vi "transition.vi"(0 "new picture in":picture, 3 "state change":bool=TRUE, 4 "game state":T1(ring), 5 "timer":dbl) -> (14 "new picture out":picture, 17 "change (of) scene":bool)   [LabVIEW 2023]
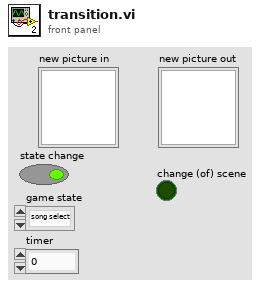
[diagram p1: front panel]
types:
  T1 = enum16{"song select", "difficulty select", "gameplay", "result"}
  T2 = cluster{"horizontal":enum16{"left", "center", "right"}, "vertical":enum16{"top", "center", "bottom"}}
  T3 = cluster{"Font Name:":string, "Size":i16, "Strikeout?":bool, "Italic?":bool, "Underline?":bool, "Outline?":bool, "Shadow?":bool, "Bold?":bool}
  T4 = enum16{"User-specified Font", "Application Font", "System Font", "Dialog Font"}
  T5 = typedef "imagedata.ctl" = cluster{"image type":i32, "image depth":i32, "image":u8[], "mask":u8[], "colors":u32[], "Rectangle":cluster{"left":i16, "top":i16, "right":i16, "bottom":i16}}
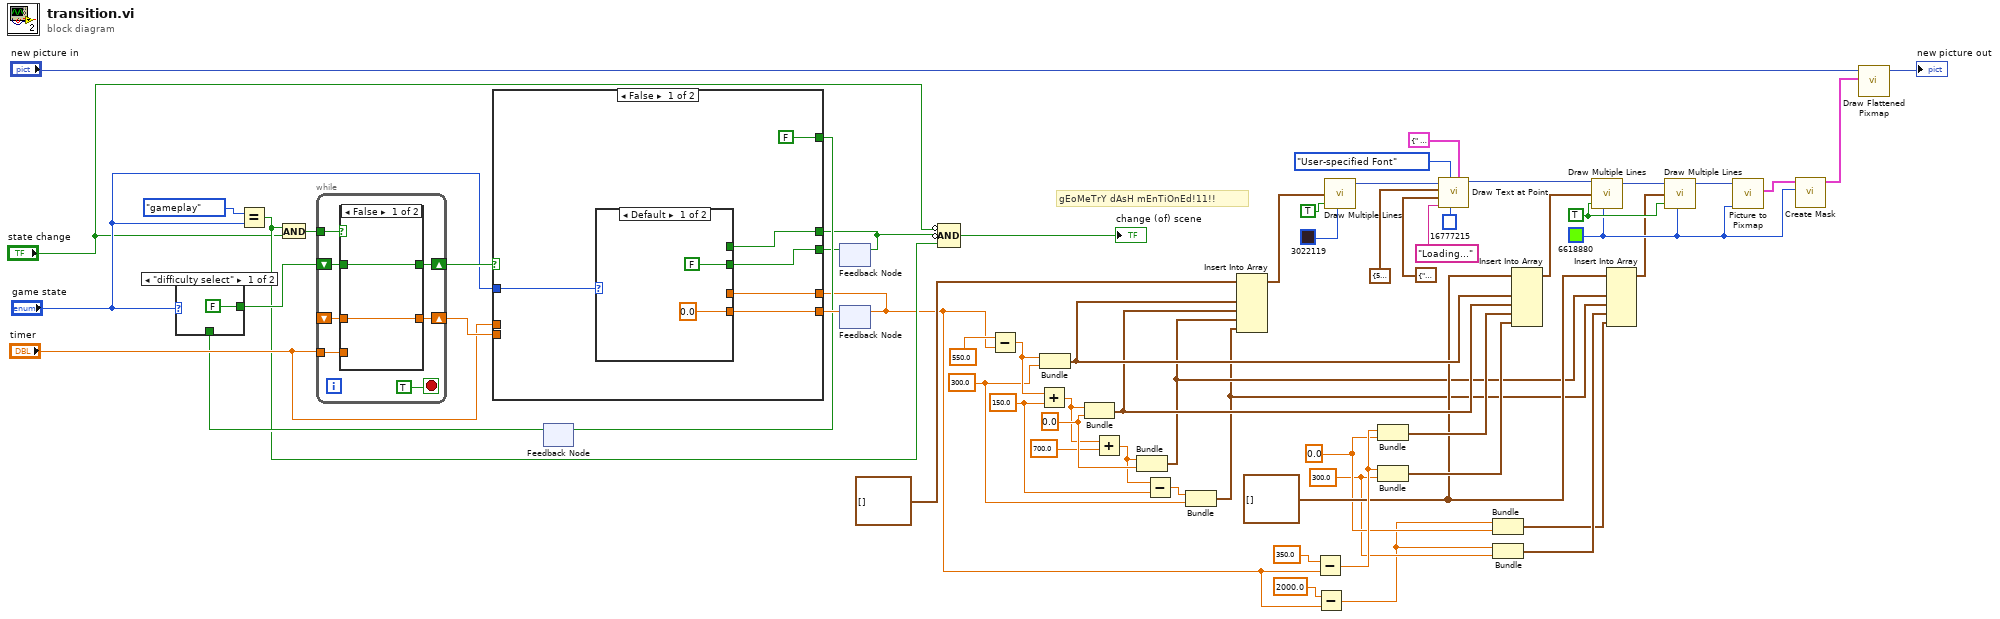
[diagram p0: block diagram]
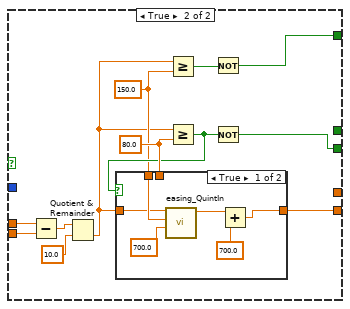
[diagram p3: hidden frame]
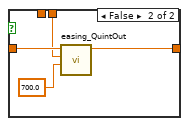
[diagram p4: hidden frame]
diagram:
  w8 = 300.0
  w9 = 0.0
  w12 = cluster{"x":i16, "y":i16}[] [] ("line endpoints")
  w14 = TRUE ("fill?(F)")
  w13 = u32 6618880 ("color(black)")
  w47 = 0.0
  w42 = 150.0
  w44 = 300.0
  # "gEoMeTrY dAsH mEnTiOnEd!11!!"
  n1 = Equal?(x=T1."gameplay" ("game state 2"), y="game state") -> (x = y?=w35:bool)
  n2 = And(x=w35, y="state change") -> (x .and. y?=w61:bool)
  n3 = feedback #1() -> (w54:bool)  [unwired: 1 in]
  n4 = case shown="\"difficulty select\"" "game state" {
    tunnel: [FALSE w64] -> w60
    tunnel: w54 -> [_ w64]
    frame "difficulty select" {
    }
    frame Default {
    }
  }
  n5 = while {
    tunnel: w61 -> [w70]
    shift-right: [w68] -> w59
    shift-left: w60 -> [w69]
    tunnel: "timer" -> [w67]
    shift-right: [w66] -> w58
    shift-left: _ -> [w65]
    stop <- TRUE stop-if-true
    n6 = case shown="False" w70 {
      selector: w70 -> [_ w74]
      tunnel: w69 -> [w72 _]
      tunnel: [w72 w74] -> w68
      tunnel: w67 -> [_ w75]
      tunnel: [w73 w75] -> w66
      tunnel: w65 -> [w73 _]
      frame False {
      }
      frame True {
      }
    }
  }
  n7 = feedback #2() -> (w32:bool)  [unwired: 1 in]
  n8 = feedback #3() -> (w6:dbl)  [unwired: 1 in]
  n9 = case shown="False" w59 {
    tunnel: w58 -> [_ w97]
    tunnel: "timer" -> [_ w96]
    tunnel: [w80 w93] -> w55
    tunnel: "game state" -> [w81 _]
    tunnel: w6 -> [w79 _]
    tunnel: [w78 w91] -> w52
    tunnel: [FALSE ("fill?(F)") w86] -> w53
    tunnel: w32 -> [w76 _]
    frame False {
      n10 = case shown="Default" w81 {
        tunnel: [0.0 w85] -> w80
        tunnel: w79 -> [_ w85]
        tunnel: [FALSE ("fill?(F)") w84] -> w78
        tunnel: w76 -> [_ w84]
        frame Default {
        }
        frame "gameplay", "result" {
        }
      }
    }
    frame True {
      w89 = 150.0 ("y")
      w92 = 80.0 ("y")
      n11 = Subtract(x=w96, y=w97) -> (x-y=w95:dbl)
      n12 = Quotient & Remainder(x=w95, y=10.0) -> (floor(x/y)=w88:dbl)  [unwired: 1 out]
      n13 = Greater Or Equal?(x=w88, y=w89) -> (x >= y?=w87:bool)
      n14 = Greater Or Equal?(x=w88, y=w92) -> (x >= y?=w90:bool)
      n15 = case shown="True" w90 {
        tunnel: [w98 w106] -> w93
        tunnel: w88 -> [w102 w105]
        tunnel: w92 -> [_ w104]
        tunnel: w89 -> [w103 _]
        frame True {
          n16 = call "easing_QuintIn.vi"("distance"=700.0, "interval (10 ms)"=w103, "time"=w102) -> ("current position"=w100:dbl)  [unwired: 8 in]
          n17 = Add(x=w100, y=700.0) -> (x+y=w98:dbl)
        }
        frame False {
          n18 = call "easing_QuintOut.vi"("distance"=700.0 ("y"), "interval (10 ms)"=w104, "time"=w105) -> ("current pos"=w106:dbl)  [unwired: 8 in]
        }
      }
      n19 = Not(x=w87) -> (.not. x?=w86:bool)
      n20 = Not(x=w90) -> (.not. x?=w91:bool)
    }
  }
  n21 = feedback-in #1(w53) -> ()
  n22 = feedback-in #2(w52) -> ()
  n23 = feedback-in #3(w55) -> ()
  n24 = Compound Arithmetic op=AND(invert "state change", invert w32, w35) -> (→"change (of) scene":bool)
  n25 = Subtract(x=550.0, y=w6) -> (x-y=w48:dbl)
  n26 = Add(x=w48, y=w42) -> (x+y=w46:dbl)
  n27 = Bundle(w48, w44) -> (w22:cluster{dbl, dbl})  [unwired: 1 in]
  n28 = Bundle(w46, w47) -> (w21:cluster{dbl, dbl})  [unwired: 1 in]
  n29 = Add(x=w46, y=700.0) -> (x+y=w41:dbl)
  n30 = Bundle(w41, w47) -> (w11:cluster{dbl, dbl})  [unwired: 1 in]
  n31 = Subtract(x=w41, y=w42) -> (x-y=w43:dbl)
  n32 = Bundle(w43, w44) -> (w10:cluster{dbl, dbl})  [unwired: 1 in]
  n33 = Insert Into Array(array=cluster{"x":i16, "y":i16}[] [] ("line endpoints"), new element #1=w22, new element #2=w21, new element #3=w11, new element #4=w10) -> (w49:cluster{"x":i16, "y":i16}[])  [unwired: 1 in]
  n34 = Subtract(x=350.0, y=w6) -> (x-y=w17:dbl)
  n35 = Subtract(x=2000.0, y=w6) -> (x-y=w5:dbl)
  n36 = call <vilib>:"Draw Multiple Lines.vi"("line endpoints"=w49, "fill?(F)"=TRUE, "color(black)"=u32 3022119) -> ("new picture"=w31:picture)  [unwired: 6 in]
  n37 = Bundle(w17, w9) -> (w20:cluster{dbl, dbl})  [unwired: 1 in]
  n38 = Bundle(w17, w8) -> (w19:cluster{dbl, dbl})  [unwired: 1 in]
  n39 = call <vilib>:"Draw Text at Point.vi"("[user-specified font]"=T3 {"Font Name:"=" ", "Size"=20, "Strikeout?"=FALSE, "Italic?"=FALSE, "Underline?"=FALSE, "Outline?"=FALSE, "Shadow?"=FALSE, "Bold?"=TRUE}, "text color(black)"=u32 16777215, "desired font(Application)"=T4."User-specified Font", "text"="Loading...", "alignment(left, top)"=T2 {"horizontal"=enum."right", "vertical"=enum."bottom"}, "origin"=cluster{"x":i16, "y":i16} {"x"=510, "y"=290}, "picture"=w31) -> ("new picture"=w24:picture)  [unwired: 3 in, 1 out]
  n40 = Bundle(w5, w9) -> (w3:cluster{dbl, dbl})  [unwired: 1 in]
  n41 = Bundle(w5, w8) -> (w4:cluster{dbl, dbl})  [unwired: 1 in]
  n42 = Insert Into Array(array=w12, new element #1=w22, new element #2=w21, new element #3=w20, new element #4=w19) -> (w23:cluster{"x":i16, "y":i16}[])  [unwired: 1 in]
  n43 = call <vilib>:"Draw Multiple Lines.vi"("picture"=w24, "line endpoints"=w23, "fill?(F)"=w14, "color(black)"=w13) -> ("new picture"=w16:picture)  [unwired: 5 in]
  n44 = Insert Into Array(array=w12, new element #1=w11, new element #2=w10, new element #3=w4, new element #4=w3) -> (w2:cluster{"x":i16, "y":i16}[])  [unwired: 1 in]
  n45 = call <vilib>:"Draw Multiple Lines.vi"("picture"=w16, "line endpoints"=w2, "fill?(F)"=w14, "color(black)"=w13) -> ("new picture"=w15:picture)  [unwired: 5 in]
  n46 = call <vilib>:"Picture to Pixmap.vi"("Background Color"=w13, "picture"=w15) -> ("image data"=w40:T5)  [unwired: 8 in, 1 out]
  n47 = call <vilib>:"Create Mask.vi"("Mask Color (Black)"=w13, "image data"=w40) -> ("image data"=w37:T5)  [unwired: 9 in]
  n48 = call <vilib>:"Draw Flattened Pixmap.vi"("image data"=w37, "picture"="new picture in") -> ("new picture"=→"new picture out":picture)  [unwired: 7 in]
